vi "CFTS-Split ID to Experimenter and Number.vi"(0 "ID":string) -> (1 "Experimenter":string, 2 "Number":i32)   [LabVIEW 2020]
uses:
  <vilib>/regexp/Match Regular Expression.xnode
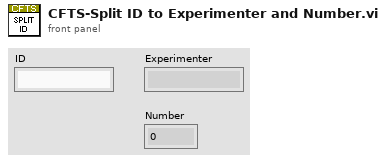
[diagram p1: front panel]
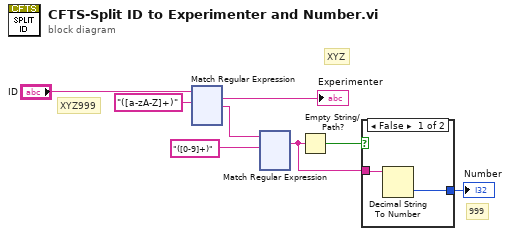
[diagram p0: block diagram]
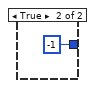
[diagram p2: hidden frame]
diagram:
  # "999"
  # "XYZ"
  # "XYZ999"
  n1 = xnode "Match Regular Expression"("input string"="ID", "regular expression"="([a-zA-Z]+)") -> ("whole match"=→"Experimenter":string, "after match"=w4:string)  [unwired: 4 in, 3 out]
  n2 = xnode "Match Regular Expression"("input string"=w4, "regular expression"="([0-9]+)") -> ("whole match"=w7:string)  [unwired: 4 in, 4 out]
  n3 = Empty String/Path?(string/path=w7) -> (empty?=w6:bool)
  n4 = case shown="False" w6 {
    tunnel: w7 -> [w10 _]
    tunnel: [w9 -1] -> w8
    frame False {
      n5 = Decimal String To Number(string=w10) -> (number=w9:i32)  [unwired: 2 in, 1 out]
    }
    frame True {
    }
  }
  "Number" <- w8
